vi "HP Loop.vi"(8 "error in (no error)":errorcluster, 11 "Timing Module in":refnum<class "Timing Module.lvclass">) -> (0 "error out":errorcluster, 3 "Timing Module out":refnum<class "Timing Module.lvclass">)   [LabVIEW 2020, in "Volatus.lvlib" / "Timing Module.lvclass"]
uses:
  Timing Module.lvclass
  C:/dev/lv20CE/relink/lv-volatus/Volatus/Module/Module.lvclass
  <vilib>/Platform/TimedLoop/XDataNode/timing_clust.ctl
  <vilib>/Platform/TimedLoop/XDataNode/nitl_modes.ctl
  <vilib>/Platform/TimedLoop/XDataNode/wakeup.ctl
  Module/Module.lvclass
  Module/Module.lvclass/Module.ctl
  <vilib>/Utility/error.llb/Error Cluster From Error Code.vi
  <vilib>/platform/TimedLoop/XDataNode/XDataNode.xnode
  Timing Module.lvclass/Timing Module.ctl
  <vilib>/Platform/TimedLoop/XDataNode/XDNodeRunTimeDep.lvlib
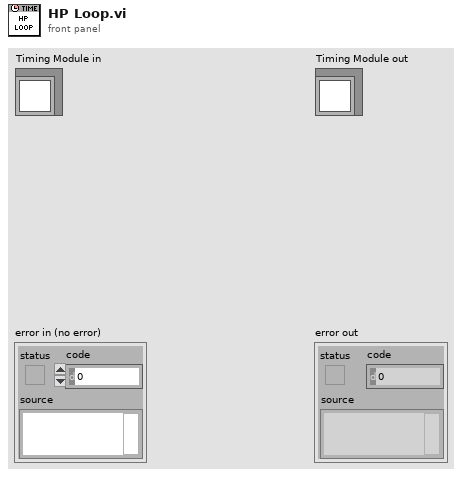
[diagram p1: front panel]
types:
  T1 = typedef "XDNodeRunTimeDep.lvlib/timing_clust.ctl" = cluster{"Expected End [f-1]":u64, "Actual End [f-1]":u64, "Finished Late? [f-1]":bool, "Expected End [i-1]":u64, "Actual End [i-1]":u64, "Finished Late? [i-1]":bool, "Expected Start [i]":u64, "Actual Start [i]":u64, "Expected Start [f]":u64, "Actual Start [f]":u64, "Source Name":string, "Structure Name":string, "Period":i64, "Deadline":i64, "Offset":i64, "Start":i64, "Priority":i32, "Timeout":i32, "Mode":T2, "Wakeup Reason":T3, "Error":errorcluster, "Source Type":string, "Secondary Source Type":string, "Global End Time":u64, "Global Start Time":u64, "Frame Duration":u64, "Iteration Duration":u64, "Assigned CPU":i32, "I/O Scan Engine Mode":u32}
  T2 = typedef "XDNodeRunTimeDep.lvlib/nitl_modes.ctl" = enum32{"No Change", "Process missed periods, maintain original phase", "Discard missed periods, maintain original phase", "Process missed periods, ignore original phase", "Discard missed periods, ignore original phase"}
  T3 = typedef "XDNodeRunTimeDep.lvlib/wakeup.ctl" = enum32{"Normal", "Aborted", "Asynchronous wakeup", "Timing source error", "Timed loop error", "Timeout"}
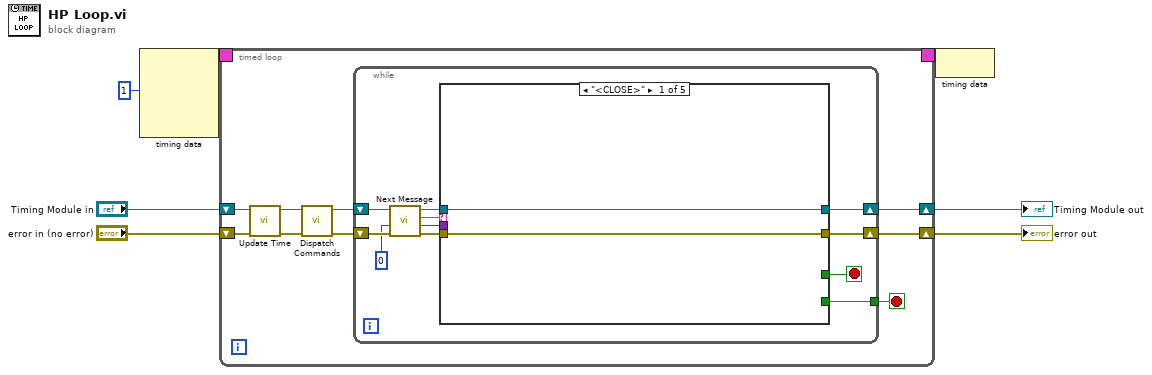
[diagram p0: block diagram]
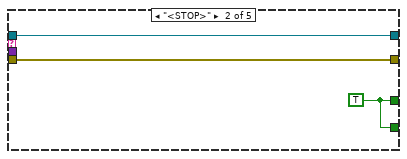
[diagram p2: hidden frame]
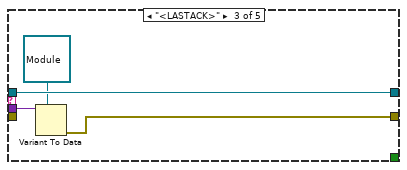
[diagram p3: hidden frame]
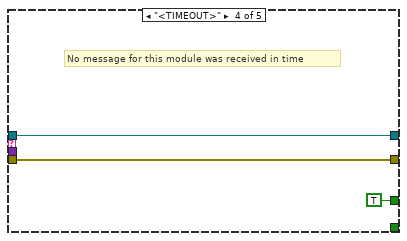
[diagram p4: hidden frame]
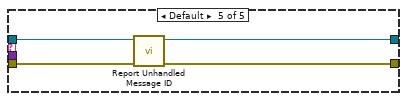
[diagram p5: hidden frame]
diagram:
  n1 = node-c288(i64 1 ("Period")) -> (w7:T1)  [unwired: 3 in]
  n2 = timed-loop {
    timing: w7 -> [_]
    timing-out: [_] -> w6
    shift-right: [w13] -> w2
    shift-left: "Timing Module in" -> [w16]
    shift-right: [w12] -> w1
    shift-left: "error in (no error)" -> [w15]
    stop <- w11 stop-if-true
    n3 = call "Update Time.vi"("error in (no error)"=w15, "Timing Module in"=w16) -> ("error out"=w14:errorcluster, "Timing Module out"=w9:refnum<class "Timing Module.lvclass">)  [unwired: 8 in]
    n4 = call "Dispatch Commands.vi"("error in (no error)"=w14, "Timing Module in"=w9) -> ("error out"=w10:errorcluster, "Timing Module out"=w8:refnum<class "Timing Module.lvclass">)  [unwired: 8 in]
    n5 = while {
      shift-right: [w22] -> w13
      shift-left: w8 -> [w27]
      shift-right: [w21] -> w12
      shift-left: w10 -> [w26]
      tunnel: [w17] -> w11
      stop <- w20 stop-if-true
      n6 = call "Next Message.vi"("error in (no error)"=w26, "Timeout ms (-1)"=0, "Module in"=w27) -> ("error out"=w25:errorcluster, "Data"=w19:variant, "ID"=w24:string, "Module out"=w23:refnum<class "Timing Module.lvclass">)  [unwired: 5 in]
      n7 = case shown="\"<CLOSE>\"" w24 {
        tunnel: w25 -> [w28 w31 _ w38 w43]
        tunnel: w23 -> [w29 w32 w36 w39 w41]
        tunnel: [w29 w32 w36 w39 w40] -> w22
        tunnel: [w28 w31 w33 w38 w42] -> w21
        tunnel: [_ w30 _ TRUE _] -> w20
        tunnel: w19 -> [_ _ w35 _ _]
        tunnel: [_ w30 _ _ _] -> w17
        frame "<CLOSE>" {
        }
        frame "<STOP>" {
          w30 = TRUE
        }
        frame "<LASTACK>" {
          n8 = Variant To Data(type=refnum<class "Module.lvclass"> refnum ("Volatus:Module"), Variant=w35) -> (error out=w33:errorcluster)  [unwired: 1 in, 1 out]
        }
        frame "<TIMEOUT>" {
          # "No message for this module was received in time"
        }
        frame Default {
          n9 = call "Report Unhandled Message ID.vi"("error in (no error)"=w43, "Module in"=w41) -> ("error out"=w42:errorcluster, "Module out"=w40:refnum<class "Timing Module.lvclass">)  [unwired: 8 in]
        }
      }
    }
  }
  "error out" <- w1
  "Timing Module out" <- w2
  n10 = node-c288(w6) -> ()
